vi "enterDriveMode.vi"(8 "error in (no error)":errorcluster, 9 "targetNumber":i16, 10 "interface object in":refnum<k20>, 11 "MotorControllerClass in":refnum<class "MotorControllerClass.lvclass">) -> (0 "error out":errorcluster, 2 "interface object out":refnum<k20>, 3 "MotorControllerClass out":refnum<class "MotorControllerClass.lvclass">, 4 "targetTorqueRes":u32, 5 "controlWord6Res":i16)   [LabVIEW 2018, in "MotorControllerClass.lvclass"]
uses:
  BMS/MotorControllerClass.lvclass
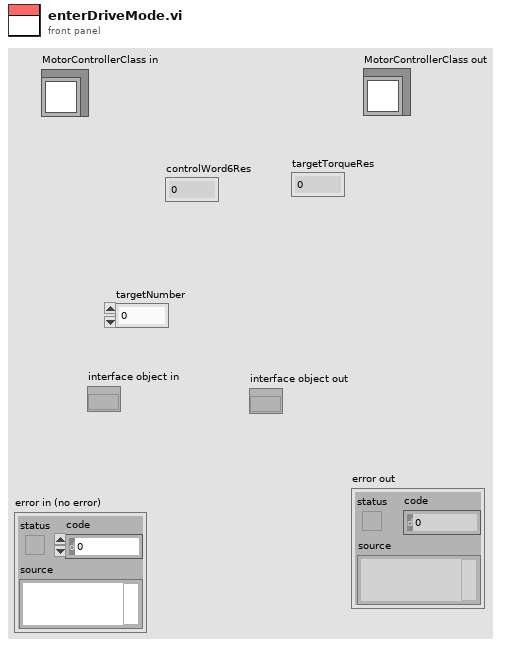
[diagram p1: front panel]
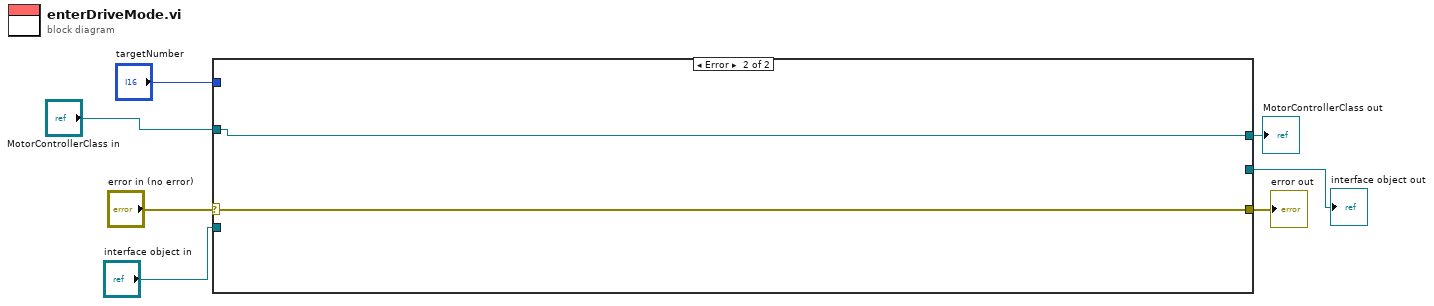
[diagram p0: block diagram]
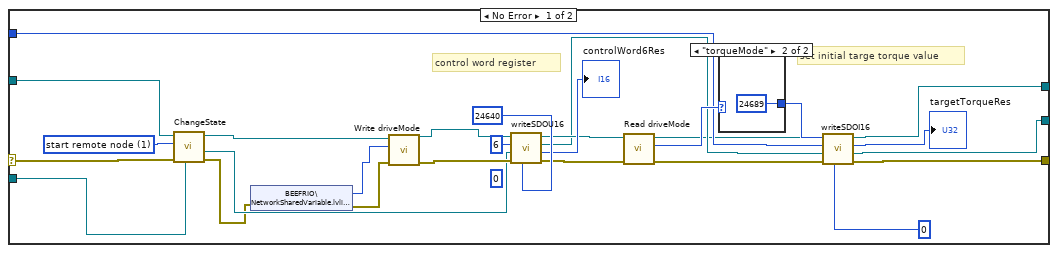
[diagram p2: hidden frame]
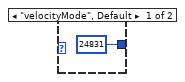
[diagram p3: hidden frame]
diagram:
  n1 = case shown="Error" "error in (no error)" {
    selector: "error in (no error)" -> [w32 w37]
    tunnel: [w14 w37] -> w6
    tunnel: [w11 w36] -> w1
    tunnel: "interface object in" -> [w31 _]
    tunnel: "targetNumber" -> [w18 _]
    tunnel: [w13 _] -> w3
    tunnel: "MotorControllerClass in" -> [w30 w36]
    frame No Error {
      w33 = u16 1 items=["start remote node"=1, "stop remote node"=2, "enter pre-operational"=128, "reset node"=129, "reset communication"=130] ("state")
      (unwired) u8 0 ("object sub-index (0)")
      # "set initial targe torque value"
      # "control word register"
      n2 = call "ChangeState.vi"("interface object in"=w31, "error in (no error)"=w32, "state"=w33, "MotorControllerClass in"=w30) -> ("error out"=w10:errorcluster, "interface object out"=w23:refnum<k20>, "MotorControllerClass out"=w29:refnum<class "MotorControllerClass.lvclass">)  [unwired: 5 in]
      n3 = shared-variable "BEEFRIO\\NetworkSharedVariable.lvlib\\driveMode"(error in=w10) -> (w8:enum16{"velocityMode", "torqueMode", ""}, error out=w9:errorcluster)
      n4 = call-dynamic "Write driveMode.vi"("error in (no error)"=w9, "driveMode"=w8, "MotorControllerClass in"=w29) -> ("error out"=w25:errorcluster, "MotorControllerClass out"=w27:refnum<class "MotorControllerClass.lvclass">)  [unwired: 7 in]
      n5 = call "writeSDOU16.vi"("object index"=u16 24640, "error in (no error)"=w25, "interface object in"=w23, "inputNumber"=u16 6, "MotorControllerClass in"=w27) -> ("error out"=w22:errorcluster, "completion code"=→"controlWord6Res":u32, "interface object out"=w17:refnum<k20>, "MotorControllerClass out"=w21:refnum<class "MotorControllerClass.lvclass">)  [unwired: 3 in]
      n6 = call-dynamic "Read driveMode.vi"("error in (no error)"=w22, "MotorControllerClass in"=w21) -> ("error out"=w16:errorcluster, "driveMode"=w20:enum16{"velocityMode", "torqueMode", ""}, "MotorControllerClass out"=w11:refnum<class "MotorControllerClass.lvclass">)  [unwired: 7 in]
      n7 = case shown="\"torqueMode\"" w20 {
        tunnel: [u16 24831 ("object index") u16 24689 ("object index")] -> w19
        frame "velocityMode", Default {
        }
        frame "torqueMode" {
        }
      }
      n8 = call "writeSDOI16.vi"("object sub-index (0)"=u8 0, "object index"=w19, "error in (no error)"=w16, "interface object in"=w17, "inputNumber"=w18, "MotorControllerClass in"=w11) -> ("error out"=w14:errorcluster, "interface object out"=w13:refnum<k20>, "completion code"=→"targetTorqueRes":u32)  [unwired: 2 in, 1 out]
    }
    frame Error {
    }
  }
  "error out" <- w6
  "interface object out" <- w3
  "MotorControllerClass out" <- w1
